vi "Excluded Names.vi"(9 "Type":T1, 10 "Rename":string) -> (2 "Valid":bool)   [LabVIEW 2020, in "_Rename.lvlib" / "_Rename.lvclass"]
uses:
  _Rename.lvclass
  _Rename.lvclass/_Rename.ctl
  _Shared/Type.ctl
  _Shared/_Shared.lvlib
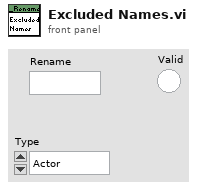
[diagram p1: front panel]
types:
  T1 = typedef "_Shared.lvlib/Type.ctl" = enum16{"Actor", "Msg"}
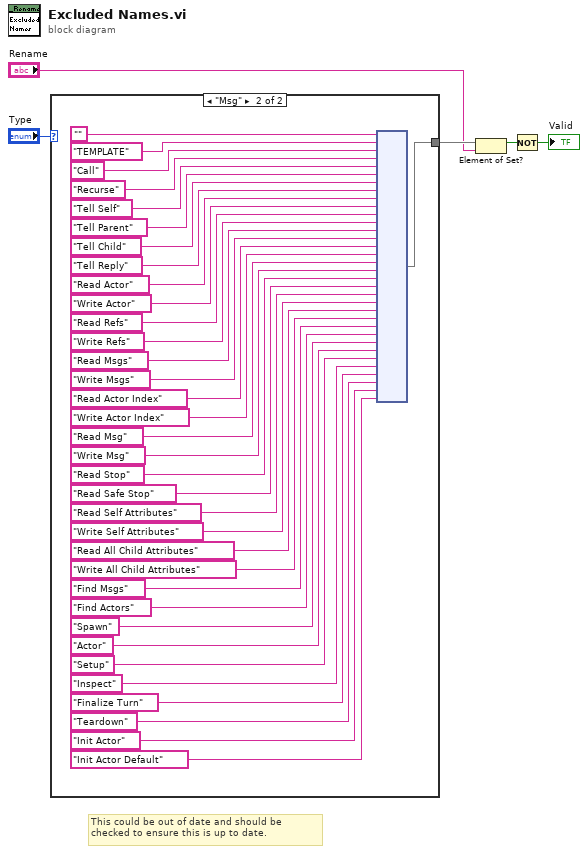
[diagram p0: block diagram]
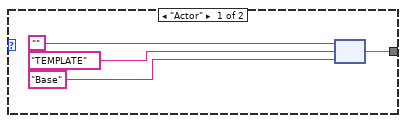
[diagram p2: hidden frame]
diagram:
  # "This could be out of date and should be checked to ensure this is up to date."
  n1 = case shown="\"Msg\"" "Type" {
    tunnel: [w7 w38] -> w2
    frame "Actor" {
      n2 = node("", "TEMPLATE", "Base") -> (w7:set{string})
    }
    frame "Msg" {
      n3 = node("", "TEMPLATE", "Call", "Recurse", "Tell Self", "Tell Parent", "Tell Child", "Tell Reply", "Read Actor", "Write Actor", "Read Refs", "Write Refs", "Read Msgs", "Write Msgs", "Read Actor Index", "Write Actor Index", "Read Msg", "Write Msg", "Read Stop", "Read Safe Stop", "Read Self Attributes", "Write Self Attributes", "Read All Child Attributes", "Write All Child Attributes", "Find Msgs", "Find Actors", "Spawn", "Actor", "Setup", "Inspect", "Finalize Turn", "Teardown", "Init Actor", "Init Actor Default") -> (w38:set{string})
    }
  }
  n4 = Element of Set?(10:"Rename", 11:w2) -> (3:w3:bool)
  n5 = Not(x=w3) -> (.not. x?=→"Valid":bool)
